vi "Spindexer Immediate Wrapper.vi"() -> ()   [LabVIEW 2019]
panel:
  in  "Setpoint":dbl
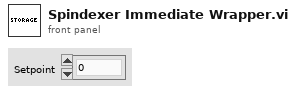
[diagram p1: front panel]
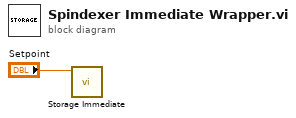
[diagram p0: block diagram]
diagram:
  n1 = call "Storage Immediate.vi"("Setpoint"="Setpoint") -> ()  [unwired: 10 in, 1 out]
